vi "Label GObject.vi"(8 "error in":errorcluster, 10 "GObject ClassName":string, 11 "GObject Reference In":refnum<vi>) -> (0 "error out":errorcluster, 1 "Terminals[]":refnum<vi>[](array[refnum]), 2 "Label":string, 3 "GObject Reference out":refnum<vi>, 5 "Excluded?":bool)   [LabVIEW 2020]
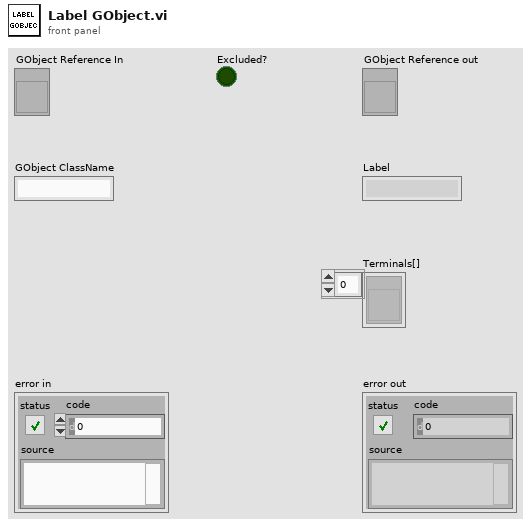
[diagram p1: front panel]
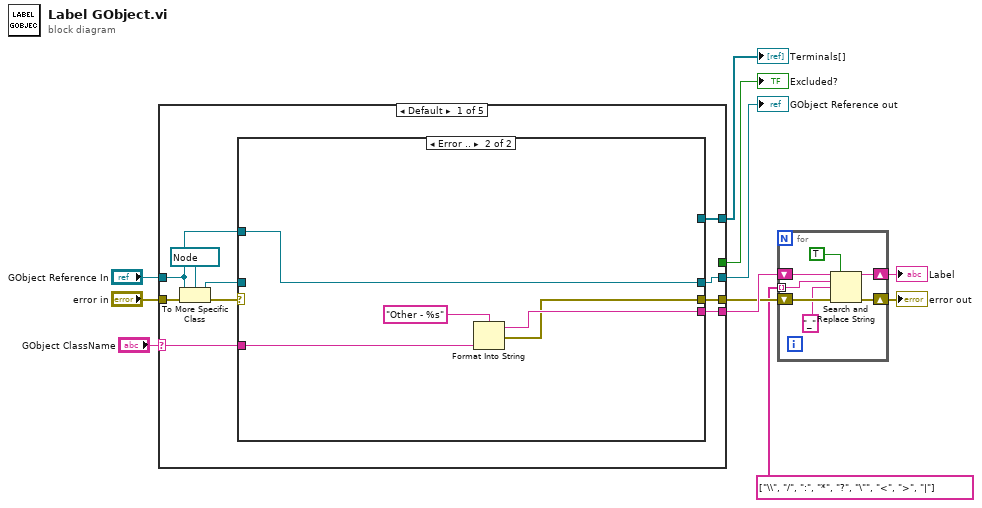
[diagram p0: block diagram]
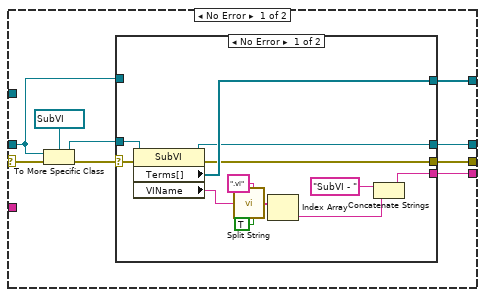
[diagram p2: hidden frame]
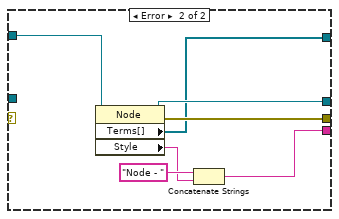
[diagram p3: hidden frame]
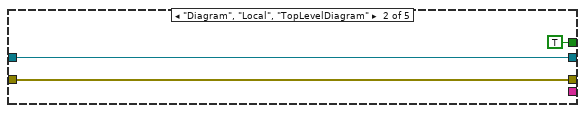
[diagram p4: hidden frame]
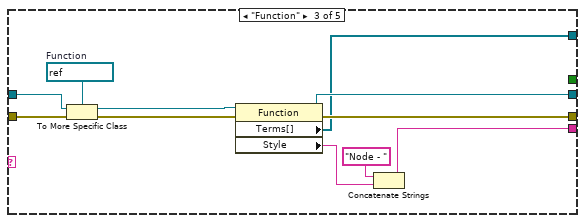
[diagram p5: hidden frame]
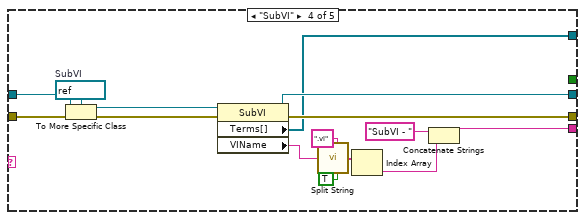
[diagram p6: hidden frame]
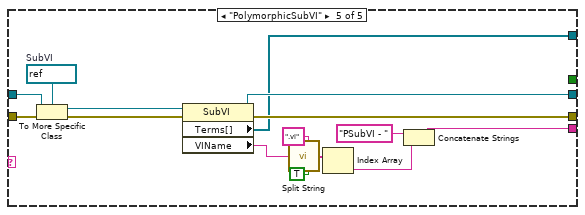
[diagram p7: hidden frame]
diagram:
  n1 = case shown="Default" "GObject ClassName" {
    selector: "GObject ClassName" -> [w20 _ _ _ _]
    tunnel: "GObject Reference In" -> [w12 w57 w64 w81 w96]
    tunnel: [w14 w57 w62 w72 w87] -> w7
    tunnel: "error in" -> [w17 w56 w65 w82 w97]
    tunnel: [w19 w56 w63 w73 w86] -> w5
    tunnel: [w21 _ w60 w76 w90] -> w6
    tunnel: [_ TRUE _ _ _] -> w8
    tunnel: [w13 _ w59 w70 w84] -> w1
    frame Default {
      n2 = To More Specific Class(target class=refnum<vi> refnum ("reference"), reference=w12, error in=w17) -> (specific class reference=w15:refnum<vi>, error out=w16:errorcluster)
      n3 = case shown="Error .." w16 {
        selector: w16 -> [w25 _]
        tunnel: [w29 w53] -> w21
        tunnel: w20 -> [_ w52]
        tunnel: [w30 w51] -> w19
        tunnel: w15 -> [w24 _]
        tunnel: [w28 w50] -> w14
        tunnel: [w27 _] -> w13
        tunnel: w12 -> [_ w50]
        frame No Error {
          n4 = To More Specific Class(target class=refnum<vi> refnum ("reference"), reference=w24, error in=w25) -> (specific class reference=w22:refnum<vi>, error out=w23:errorcluster)
          n5 = case shown="No Error" w23 {
            selector: w23 -> [w36 _]
            tunnel: [w32 w47] -> w30
            tunnel: [w31 w46] -> w29
            tunnel: [w33 w45] -> w28
            tunnel: [w34 w44] -> w27
            tunnel: w24 -> [_ w43]
            tunnel: w22 -> [w35 _]
            frame No Error {
              n6 = property on="Property Node" class="SubVI"(reference=w35, error in=w36) -> (reference out=w33:refnum<vi>, error out=w32:errorcluster, "Terms[]"=w34:refnum<vi>[], "VIName"=w38:string)
              n7 = call <vilib>:"Split String.vi"("Ignore Case? (false)"=TRUE, "Split Pattern"=".vi", "Input String"=w38) -> ("Split String"=w41:string[])  [unwired: 4 in]
              n8 = Index Array(array=w41) -> (element=w39:string)  [unwired: 1 in]
              n9 = Concatenate Strings("SubVI - " ("format string"), w39) -> (w31:string)
            }
            frame Error {
              n10 = property class="Node"(reference=w43) -> (reference out=w45:refnum<vi>, error out=w47:errorcluster, "Terms[]"=w44:refnum<vi>[], "Style"=w48:string)  [unwired: 1 in]
              n11 = Concatenate Strings("Node - " ("format string"), w48) -> (w46:string)
            }
          }
        }
        frame Error {
          n12 = Format Into String(format string="Other - %s", w52) -> (resulting string=w53:string, error out=w51:errorcluster)  [unwired: 2 in]
        }
      }
    }
    frame "Diagram", "Local", "TopLevelDiagram" {
    }
    frame "Function" {
      w68 = refnum<vi> refnum  # Function
      n13 = To More Specific Class(target class=w68, reference=w64, error in=w65) -> (specific class reference=w67:refnum<vi>, error out=w66:errorcluster)
      n14 = property on="Property Node" class="Function"(reference=w67, error in=w66) -> (reference out=w62:refnum<vi>, error out=w63:errorcluster, "Terms[]"=w59:refnum<vi>[], "Style"=w58:string)
      n15 = Concatenate Strings("Node - " ("format string"), w58) -> (w60:string)
    }
    frame "SubVI" {
      w83 = refnum<vi> refnum  # SubVI
      n16 = To More Specific Class(target class=w83, reference=w81, error in=w82) -> (specific class reference=w74:refnum<vi>, error out=w75:errorcluster)
      n17 = property on="Property Node" class="SubVI"(reference=w74, error in=w75) -> (reference out=w72:refnum<vi>, error out=w73:errorcluster, "Terms[]"=w70:refnum<vi>[], "VIName"=w71:string)
      n18 = call <vilib>:"Split String.vi"("Ignore Case? (false)"=TRUE, "Split Pattern"=".vi", "Input String"=w71) -> ("Split String"=w79:string[])  [unwired: 4 in]
      n19 = Index Array(array=w79) -> (element=w77:string)  [unwired: 1 in]
      n20 = Concatenate Strings("SubVI - " ("format string"), w77) -> (w76:string)
    }
    frame "PolymorphicSubVI" {
      w98 = refnum<vi> refnum  # SubVI
      n21 = To More Specific Class(target class=w98, reference=w96, error in=w97) -> (specific class reference=w88:refnum<vi>, error out=w89:errorcluster)
      n22 = property on="Property Node" class="SubVI"(reference=w88, error in=w89) -> (reference out=w87:refnum<vi>, error out=w86:errorcluster, "Terms[]"=w84:refnum<vi>[], "VIName"=w85:string)
      n23 = call <vilib>:"Split String.vi"("Ignore Case? (false)"=TRUE, "Split Pattern"=".vi", "Input String"=w85) -> ("Split String"=w94:string[])  [unwired: 4 in]
      n24 = Index Array(array=w94) -> (element=w91:string)  [unwired: 1 in]
      n25 = Concatenate Strings("PSubVI - " ("format string"), w91) -> (w90:string)
    }
  }
  "Excluded?" <- w8
  "GObject Reference out" <- w7
  "Terminals[]" <- w1
  n26 = for {
    shift-right: [w103] -> w3
    shift-left: w5 -> [w104]
    shift-right: [w102] -> w4
    shift-left: w6 -> [w105]
    tunnel: string[] ["\\", "/", ":", "*", "?", "\"", "<", ">", "|"] ("String") -> [w101] mode=indexing
    n27 = Search and Replace String(replace all?=TRUE ("replace all? (F)"), input string=w105, search string=w101, replace string="_" ("replace string (\"\")"), error in=w104) -> (result string=w102:string, error out=w103:errorcluster)  [unwired: 3 in, 2 out]
  }
  "error out" <- w3
  "Label" <- w4
